vi "cluster_v01.vi"() -> ()   [LabVIEW 2009]
panel:
  out "XY Graph":cluster{i32[], dbl[]}(graph)
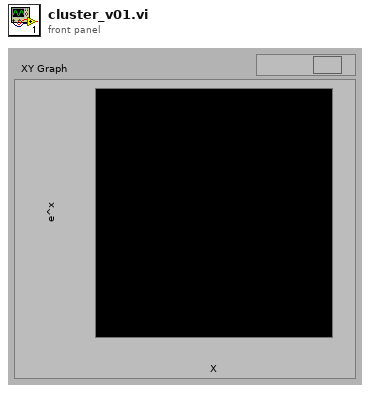
[diagram p1: front panel]
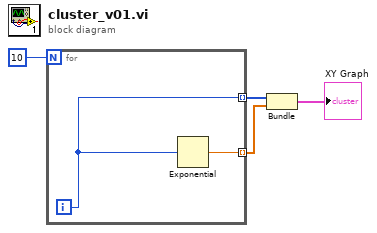
[diagram p0: block diagram]
diagram:
  n1 = for {
    N: 10 -> [_]
    tunnel: [w5] -> w3 mode=indexing
    tunnel: [w6] -> w2 mode=indexing
    i -> [w5]
    n2 = Exponential(1:w5) -> (0:w6:dbl)
  }
  n3 = Bundle(w3, w2) -> (→"XY Graph":cluster{i32[], dbl[]})  [unwired: 1 in]
